vi "Stream_5channels.vi"() -> ()   [LabVIEW 2014]
uses:
  <vilib>/FPGAPlugInAG/PXI-7852R/niLvFpga_Open_PXI-7852R.vi
  <vilib>/rvi/interface/common/dynamic/niFpgaDynamicAddResources.vi
  <vilib>/Utility/error.llb/Error Cluster From Error Code.vi
  <vilib>/rvi/errors/niLvFpgaAdjustHostInterfaceError.vi
  <vilib>/measure/maspectr.llb/FFT Power Spectrum and PSD for 1 Chan.vi
  <vilib>/FPGAPlugInAG/Dynamic/niLvFpga_Close_Dynamic.vi
  <vilib>/rvi/interface/nirviOpenFPGA/nirviOpenFPGA.xnode
  FPGA Bitfiles/MilitaruDAQ_FPGATarget_Acquisition5chan_eJYq7ojEddM.lvbitx
  Acquisition_5channels.vi
  <vilib>/rvi/interface/nirviReadWriteControl/nirviReadWriteControl.xnode
  <vilib>/rvi/interface/nirviMethod/nirviMethod.xnode
  <vilib>/rvi/interface/nirviCloseFPGA/nirviCloseFPGA.xnode
  <vilib>/FPGAPlugInAG/Dynamic/niLvFpga_ReadFifo_Dynamic.vi
  <vilib>/rvi/errors/niLvFpgaMergeErrorWithErrorCode.vi
  NiFpgaLv.dll
  <vilib>/rvi/interface/Simulation/niFpgaSimulationCallBeginRW.vi
  <vilib>/measure/NI_MAPro.lvlib
panel:
  in  "Number of\n Elements":u32
  out "Elements Remaining":u32
  in  "Sampling ticks":u32
  out "Z-balanced 2":waveform(i16)(graph) caption="Dynamic Data Type"
  in  "dB On (F) Z-balanced":bool
  in  "Z-balanced":T1={"averaging mode"=enum."No averaging", "weighting mode"=enum."Exponential", "number of averages"=10} {"number of averages" min=1}
  out "PSD Z-balanced":cluster{"f0":dbl, "df":dbl, "magnitude":dbl[]}(graph) caption="Dynamic Data Type"
  out "X 2":waveform(i16)(graph) caption="Dynamic Data Type"
  in  "dB On (F) X":bool
  in  "X":T1={"averaging mode"=enum."No averaging", "weighting mode"=enum."Exponential", "number of averages"=10} {"number of averages" min=1}
  out "PSD X":cluster{"f0":dbl, "df":dbl, "magnitude":dbl[]}(graph) caption="Dynamic Data Type"
  out "Y 2":waveform(i16)(graph) caption="Dynamic Data Type"
  in  "dB On (F) Y":bool
  in  "Y":T1={"averaging mode"=enum."No averaging", "weighting mode"=enum."Exponential", "number of averages"=10} {"number of averages" min=1}
  out "PSD Y":cluster{"f0":dbl, "df":dbl, "magnitude":dbl[]}(graph) caption="Dynamic Data Type"
  out "Z-unbalanced 2":waveform(i16)(graph) caption="Dynamic Data Type"
  in  "dB On (F)Z-unbalanced":bool
  in  "Z-unbalanced":T1={"averaging mode"=enum."No averaging", "weighting mode"=enum."Exponential", "number of averages"=10} {"number of averages" min=1}
  out "PSD Z-unbalanced":cluster{"f0":dbl, "df":dbl, "magnitude":dbl[]}(graph) caption="Dynamic Data Type"
  in  "AOM update\nrate (ticks)":u32
  in  "AOM-DC":i16
  out "Data-sampling (kHz)":dbl
  out "Z-unbalanced\n (FPGA)":bool
  out "Z-balanced\n (FPGA)":bool
  out "FIFO X\n (FPGA)":bool
  out "FIFO Z-unbalanced\n (FPGA)":bool
  out "FIFO Y\n (FPGA)":bool
  out "FIFO Z-balanced\n (FPGA)":bool
  out "data FIFO\n (FPGA)":bool
  out "AOM update (FPGA)":bool
  out "FIFO-acquisition\n (FPGA)":bool
  out "Y (FPGA)":bool
  out "X (FPGA)":bool
  out "Acquisition\n Timeout (FPGA)":bool
  out "DC acquisition (FPGA)":bool
  out "DC FIFO (FPGA)":bool
  out "DC elements remaining":u32
  in  "DC Elements":u32
  in  "DC sampling":u32
  out "DC":waveform(i16)(graph) caption="Dynamic Data Type"
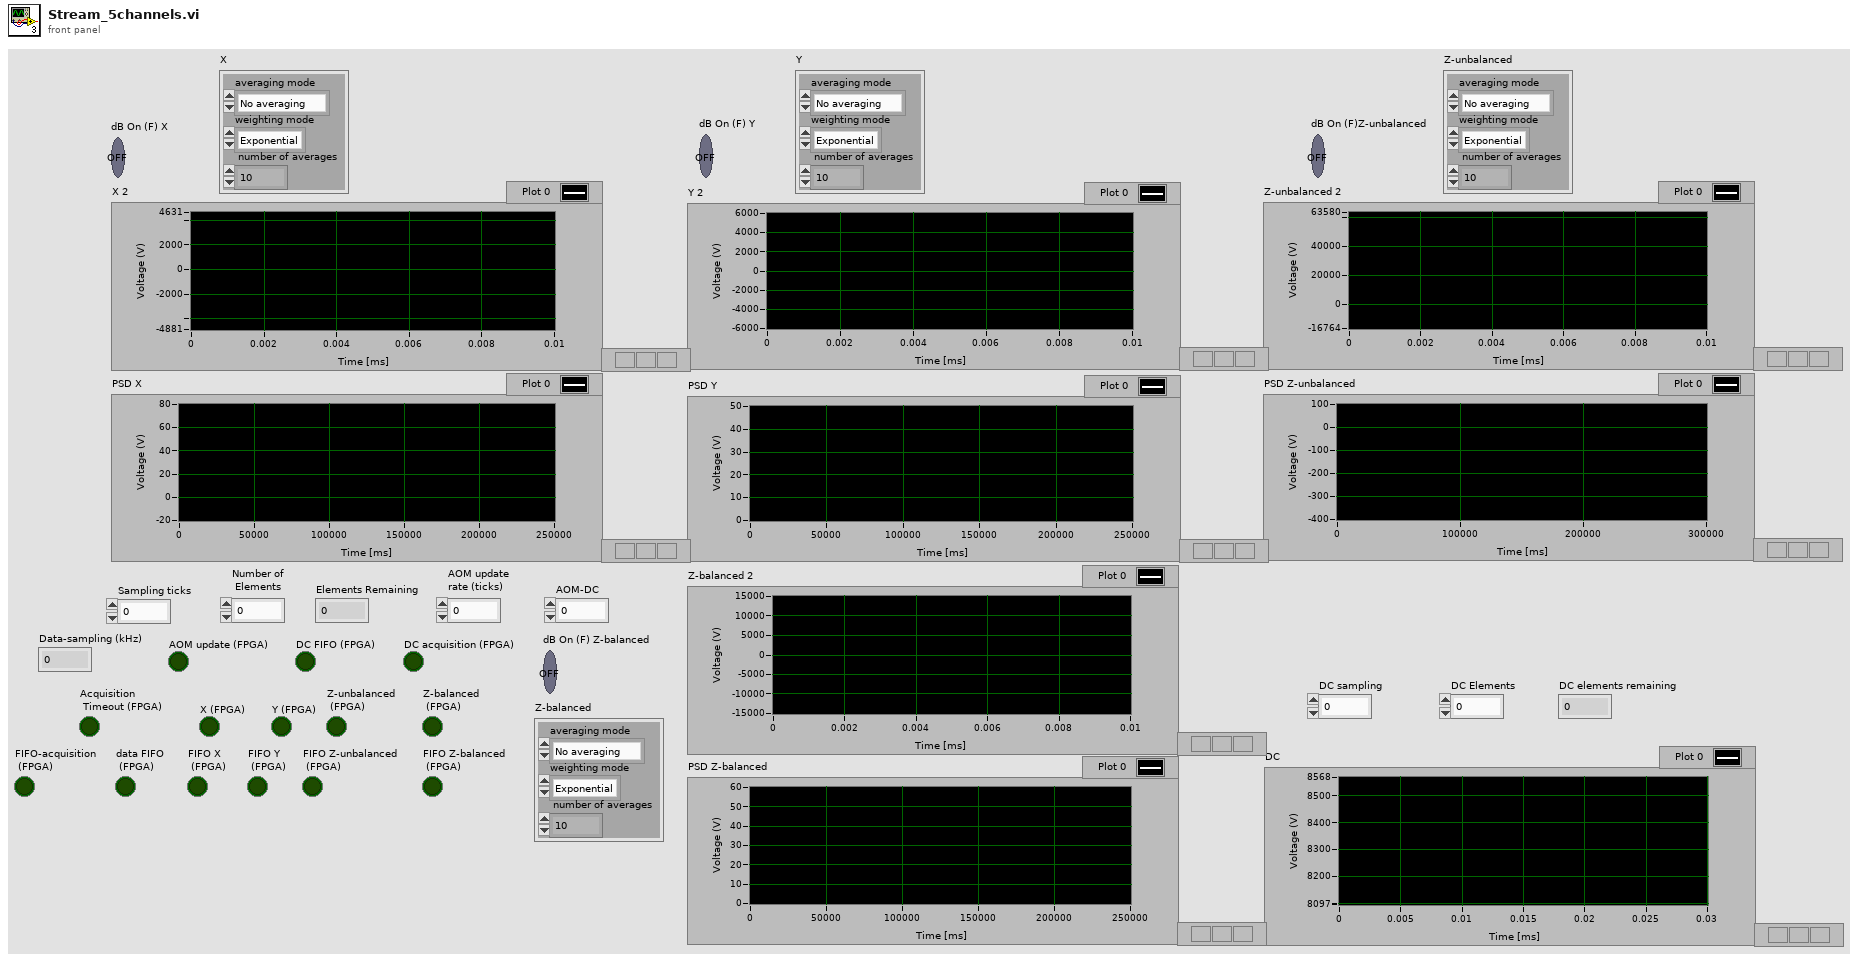
[diagram p1: front panel]
types:
  T1 = cluster{"averaging mode":enum16{"No averaging", "Vector averaging", "RMS averaging", "Peak hold"}, "weighting mode":enum16{"Linear", "Exponential"}, "number of averages":u32}
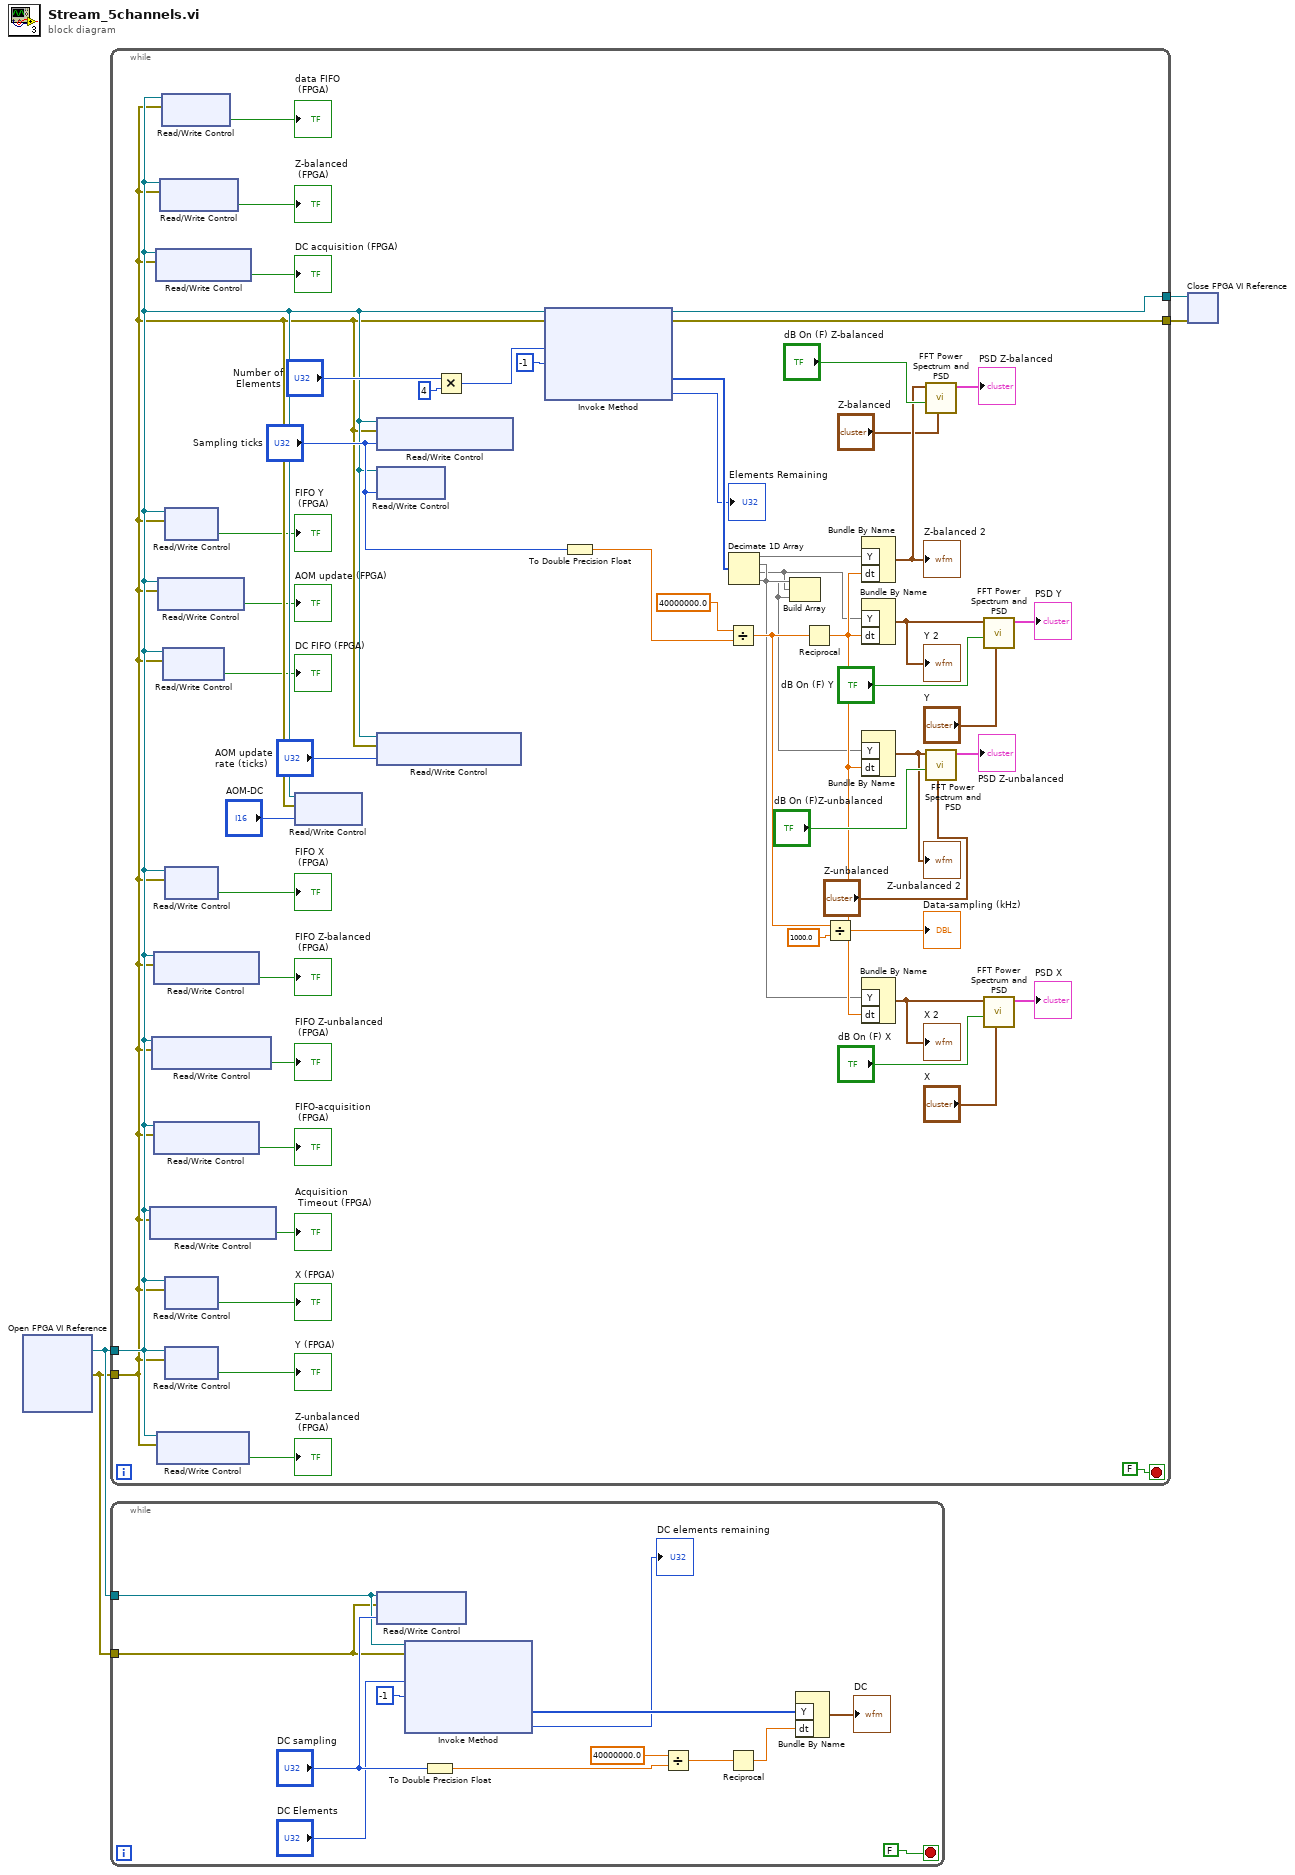
[diagram p0: block diagram]
diagram:
  n1 = xnode "Open FPGA VI Reference"() -> ("FPGA VI Reference Out"=w4:refnum<k20>, "error out"=w3:errorcluster)  [unwired: 2 in]
  n2 = while {
    tunnel: w4 -> [w29]
    tunnel: w3 -> [w28]
    tunnel: [w52] -> w2
    tunnel: [w51] -> w1
    stop <- FALSE stop-if-true
    n3 = xnode "Read/Write Control"("FPGA VI Reference In"=w29, "error in"=w28) -> ("Acquisition Timeout"=→"Acquisition\n Timeout (FPGA)":bool)  [unwired: 2 out]
    n4 = xnode "Read/Write Control"("FPGA VI Reference In"=w29, "error in"=w28) -> ("FIFO Z-unbalanced"=→"FIFO Z-unbalanced\n (FPGA)":bool)  [unwired: 2 out]
    n5 = xnode "Read/Write Control"("FPGA VI Reference In"=w29, "error in"=w28) -> ("FIFO Z-balanced"=→"FIFO Z-balanced\n (FPGA)":bool)  [unwired: 2 out]
    n6 = xnode "Read/Write Control"("FPGA VI Reference In"=w29, "error in"=w28) -> ("FIFO-acquisition"=→"FIFO-acquisition\n (FPGA)":bool)  [unwired: 2 out]
    n7 = xnode "Read/Write Control"("FPGA VI Reference In"=w29, "error in"=w28) -> ("DC acquisition"=→"DC acquisition (FPGA)":bool)  [unwired: 2 out]
    n8 = xnode "Read/Write Control"("FPGA VI Reference In"=w29, "error in"=w28) -> ("Z-unbalanced"=→"Z-unbalanced\n (FPGA)":bool)  [unwired: 2 out]
    n9 = xnode "Read/Write Control"("FPGA VI Reference In"=w29, "error in"=w28) -> ("AOM update"=→"AOM update (FPGA)":bool)  [unwired: 2 out]
    n10 = xnode "Read/Write Control"("FPGA VI Reference In"=w29, "error in"=w28) -> ("Z-balanced"=→"Z-balanced\n (FPGA)":bool)  [unwired: 2 out]
    n11 = xnode "Read/Write Control"("FPGA VI Reference In"=w29, "error in"=w28) -> ("data FIFO"=→"data FIFO\n (FPGA)":bool)  [unwired: 2 out]
    n12 = xnode "Read/Write Control"("FPGA VI Reference In"=w29, "error in"=w28) -> ("DC FIFO"=→"DC FIFO (FPGA)":bool)  [unwired: 2 out]
    n13 = xnode "Read/Write Control"("FPGA VI Reference In"=w29, "error in"=w28) -> ("FIFO Y"=→"FIFO Y\n (FPGA)":bool)  [unwired: 2 out]
    n14 = xnode "Read/Write Control"("FPGA VI Reference In"=w29, "error in"=w28) -> ("FIFO X"=→"FIFO X\n (FPGA)":bool)  [unwired: 2 out]
    n15 = xnode "Read/Write Control"("FPGA VI Reference In"=w29, "error in"=w28) -> ("X"=→"X (FPGA)":bool)  [unwired: 2 out]
    n16 = xnode "Read/Write Control"("FPGA VI Reference In"=w29, "error in"=w28) -> ("Y"=→"Y (FPGA)":bool)  [unwired: 2 out]
    n17 = xnode "Read/Write Control"("FPGA VI Reference In"=w29, "error in"=w28, "AOM-DC"="AOM-DC") -> ()  [unwired: 2 out]
    n18 = xnode "Read/Write Control"("FPGA VI Reference In"=w29, "error in"=w28, "Interleaving  Sampling"="Sampling ticks") -> ()  [unwired: 2 out]
    n19 = xnode "Read/Write Control"("FPGA VI Reference In"=w29, "Sampling"="Sampling ticks") -> ()  [unwired: 1 in, 2 out]
    n20 = xnode "Read/Write Control"("FPGA VI Reference In"=w29, "error in"=w28, "AOM update rate (ticks)"="AOM update\nrate (ticks)") -> ()  [unwired: 2 out]
    n21 = Multiply(x="Number of\n Elements", y=u32 4) -> (x*y=w55:u32)
    n22 = xnode "Invoke Method"("FPGA VI Reference In"=w29, "error in"=w28, "Number of Elements"=w55, "Timeout (ms)"=-1) -> ("FPGA VI Reference Out"=w52:refnum<k20>, "error out"=w51:errorcluster, "Data"=w54:i16[], "Elements Remaining"=→"Elements Remaining":u32)
    n23 = To Double Precision Float(number="Sampling ticks") -> (double precision float=w50:dbl)
    n24 = Divide(x=40000000.0, y=w50) -> (x/y=w12:dbl)
    n25 = Decimate 1D Array(w54) -> (w7:i16[], w9:i16[], w6:i16[], w8:i16[])
    n26 = Build Array(w9, w6, w8) -> ()  [unwired: 1 out]
    n27 = Reciprocal(x=w12) -> (1/x=w11:dbl)
    n28 = Divide(x=w12, y=1000.0) -> (x/y=→"Data-sampling (kHz)":dbl)
    n29 = Bundle By Name ("Build Waveform")("Y"=w7, "dt"=w11) -> (w47:waveform(i16))  [unwired: 1 in]
    "Z-balanced 2" <- w47
    n30 = Bundle By Name ("Build Waveform")("Y"=w6, "dt"=w11) -> (w37:waveform(i16))  [unwired: 1 in]
    "Y 2" <- w37
    n31 = Bundle By Name ("Build Waveform")("Y"=w8, "dt"=w11) -> (w33:waveform(i16))  [unwired: 1 in]
    "Z-unbalanced 2" <- w33
    n32 = Bundle By Name ("Build Waveform")("Y"=w9, "dt"=w11) -> (w41:waveform(i16))  [unwired: 1 in]
    "X 2" <- w41
    n33 = call-poly <vilib>:"FFT Power Spectrum and PSD.vi"("averaging parameters"="Z-balanced", "dB On (F)"="dB On (F) Z-balanced", "time signal"=w47) -> ("Power Spectrum / PSD"=→"PSD Z-balanced":cluster{"f0":dbl, "df":dbl, "magnitude":dbl[]})  [unwired: 5 in, 3 out]
    n34 = call-poly <vilib>:"FFT Power Spectrum and PSD.vi"("averaging parameters"="Z-unbalanced", "dB On (F)"="dB On (F)Z-unbalanced", "time signal"=w33) -> ("Power Spectrum / PSD"=→"PSD Z-unbalanced":cluster{"f0":dbl, "df":dbl, "magnitude":dbl[]})  [unwired: 5 in, 3 out]
    n35 = call-poly <vilib>:"FFT Power Spectrum and PSD.vi"("averaging parameters"="Y", "dB On (F)"="dB On (F) Y", "time signal"=w37) -> ("Power Spectrum / PSD"=→"PSD Y":cluster{"f0":dbl, "df":dbl, "magnitude":dbl[]})  [unwired: 5 in, 3 out]
    n36 = call-poly <vilib>:"FFT Power Spectrum and PSD.vi"("averaging parameters"="X", "dB On (F)"="dB On (F) X", "time signal"=w41) -> ("Power Spectrum / PSD"=→"PSD X":cluster{"f0":dbl, "df":dbl, "magnitude":dbl[]})  [unwired: 5 in, 3 out]
  }
  n37 = while {
    tunnel: w4 -> [w62]
    tunnel: w3 -> [w61]
    stop <- FALSE stop-if-true
    n38 = xnode "Read/Write Control"("FPGA VI Reference In"=w62, "error in"=w61, "DC-Sampling"="DC sampling") -> ()  [unwired: 2 out]
    n39 = xnode "Invoke Method"("FPGA VI Reference In"=w62, "error in"=w61, "Number of Elements"="DC Elements", "Timeout (ms)"=-1) -> ("Data"=w67:i16[], "Elements Remaining"=→"DC elements remaining":u32)  [unwired: 2 out]
    n40 = To Double Precision Float(number="DC sampling") -> (double precision float=w68:dbl)
    n41 = Divide(x=40000000.0, y=w68) -> (x/y=w60:dbl)
    n42 = Reciprocal(x=w60) -> (1/x=w59:dbl)
    n43 = Bundle By Name ("Build Waveform")("Y"=w67, "dt"=w59) -> (→"DC":waveform(i16))  [unwired: 1 in]
  }
  n44 = xnode "Close FPGA VI Reference"("FPGA VI Reference In"=w2, "error in"=w1) -> ()  [unwired: 1 out]
